vi "Periodic Message Generator.vi"(0 "J1939 Cluster":T4, 1 "Scale Ref":T2, 2 "Data Ref":T1, 5 "Output Array":T3[](array[typedef]) {"Identifier" format="%08x"}, 7 "Timeouts":T5[](array[typedef]) {"Arb ID" format="%.0x"}, 11 "error in":errorcluster) -> (4 "J1939 Cluster Out":T4, 6 "Output Array":T3[](array[typedef]) {"Identifier" format="%08x"}, 8 "Empty?":bool, 15 "error out":errorcluster)   [LabVIEW 2015, in "J1939 Addon Engine.lvlib"]
uses:
  J1939 Addon Engine.lvlib
  SubVIs/Periodic Message Generator Cluster.ctl
  Shared/J1939 Utilities/Types/CAN Outgoing Message Cluster.ctl
  Types/Setup Information Cluster.ctl
  <vilib>/xnet/xnet.llb/XNET Frame CAN.ctl
  <vilib>/xnet/xnet.llb/XNET Frame Type CAN.ctl
  Types/Conversion Lookup Table Reference.ctl
  Types/Data Lookup Table Reference.ctl
  Types/Datatable Lookup DVR.ctl
  Conversion Lookup Table Get Conversion Parameter.vi
  Data Lookup Table Get Signals (Range).vi
  <vilib>/xnet/xnet.llb/XNET Convert.vi
  <vilib>/xnet/xnet.llb/XNET Convert (Signal to Frame Raw).vi
  Data Lookup Table.vi
  Conversion Lookup Table.vi
  Shared/J1939 Utilities/J1939 Utilities.lvlib
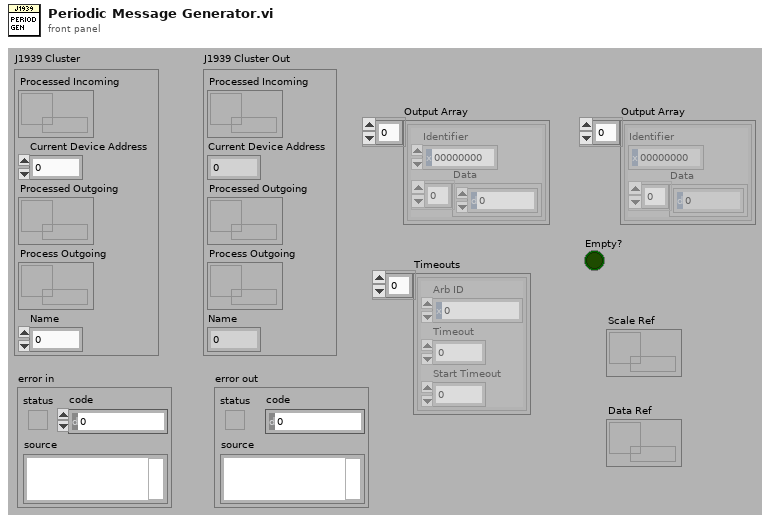
[diagram p1: front panel]
types:
  T1 = typedef "J1939 Addon Engine.lvlib/Data Lookup Table Reference.ctl" = refnum<data-value>
  T2 = typedef "J1939 Addon Engine.lvlib/Conversion Lookup Table Reference.ctl" = refnum<data-value>
  T3 = typedef "J1939 Addon Shared.lvlib/J1939 Utilities.lvlib/CAN Outgoing Message Cluster.ctl" = cluster{"Identifier":u32, "Data":u8[]}
  T4 = typedef "J1939 Addon Engine.lvlib/Setup Information Cluster.ctl" = cluster{"Processed Incoming":refnum<queue>, "Current Device Address":u8, "Processed Outgoing":refnum<queue>, "Process Outgoing":refnum<queue>, "Name":u64}
  T5 = typedef "J1939 Addon Engine.lvlib/Periodic Message Generator Cluster.ctl" = cluster{"Arb ID":u32, "Timeout":u32, "Start Timeout":u32}
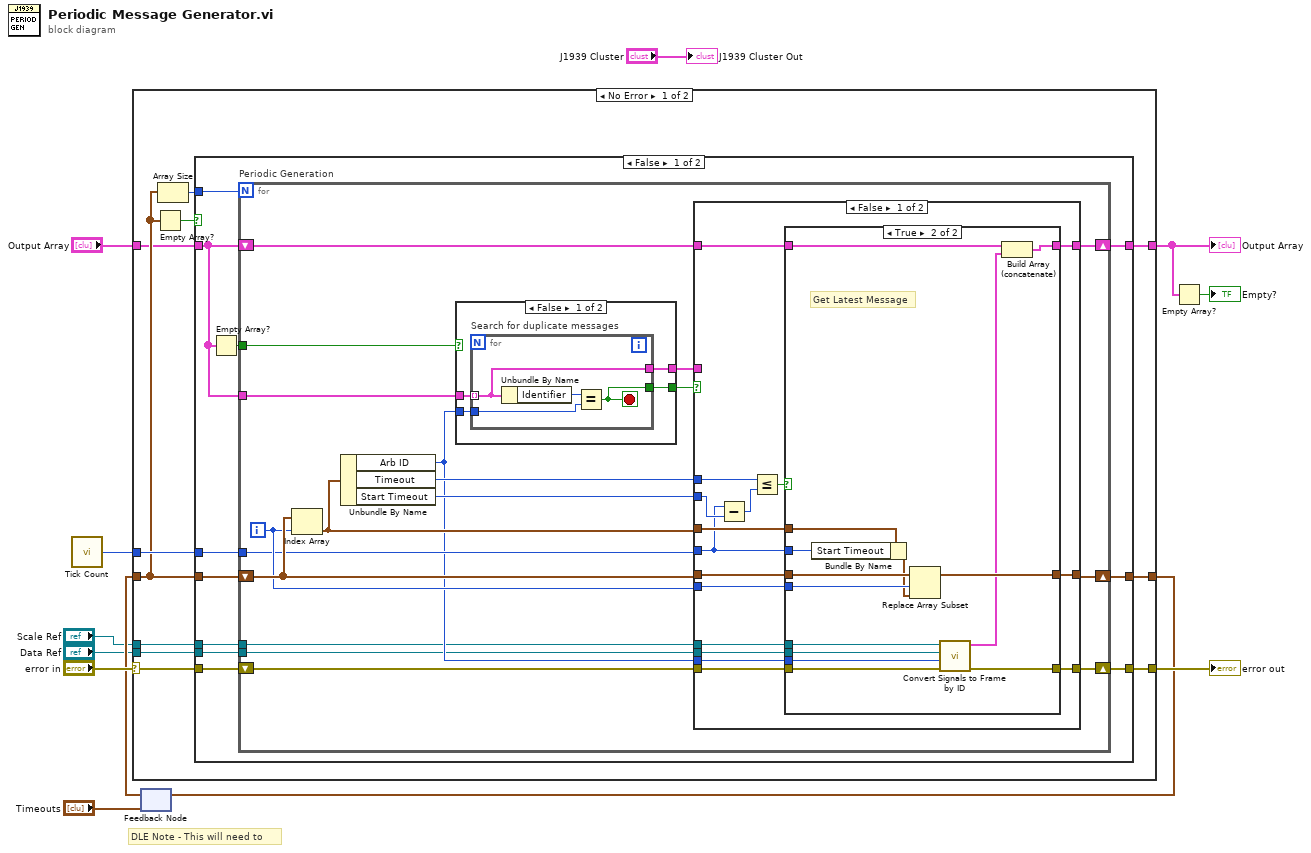
[diagram p0: block diagram]
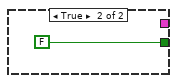
[diagram p2: hidden frame]
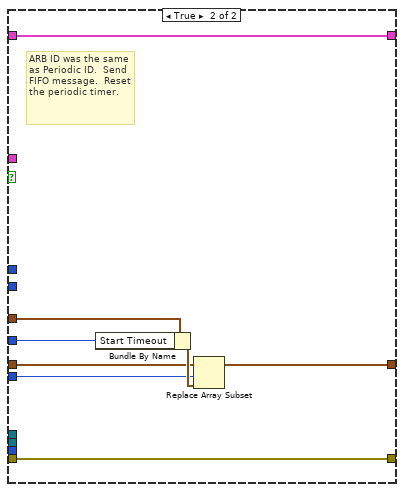
[diagram p4: hidden frame]
diagram:
  # "DLE Note - This will need to"
  n1 = call "Tick Count"() -> ("Tick Count(mSec)"=w10:u32)
  n2 = feedback #1("Timeouts") -> (w3:T5[])
  n3 = case shown="No Error" "error in" {
    selector: "error in" -> [w16 w108]
    tunnel: w3 -> [w20 w107]
    tunnel: [w22 w106] -> w6
    tunnel: [w15 w108] -> w11
    tunnel: w10 -> [w21 _]
    tunnel: [w18 w107] -> w9
    tunnel: "Output Array" -> [w17 w106]
    tunnel: "Scale Ref" -> [w14 _]
    tunnel: "Data Ref" -> [w13 _]
    frame No Error {
      n4 = Empty Array?(array=w20) -> (empty?=w19:bool)
      n5 = Array Size(array=w20) -> (size(s)=w23:i32)
      n6 = case shown="False" w19 {
        tunnel: w23 -> [w34 _]
        tunnel: [w30 w105] -> w22
        tunnel: w21 -> [w32 _]
        tunnel: w17 -> [w27 w105]
        tunnel: w20 -> [w33 w104]
        tunnel: [w31 w104] -> w18
        tunnel: w16 -> [w29 w103]
        tunnel: [w28 w103] -> w15
        tunnel: w14 -> [w25 _]
        tunnel: w13 -> [w24 _]
        frame False {
          n7 = Empty Array?(array=w27) -> (empty?=w26:bool)
          n8 = for "Periodic Generation" {
            N: w34 -> [_]
            tunnel: w32 -> [w44]
            shift-right: [w51] -> w30
            shift-left: w27 -> [w52]
            shift-right: [w48] -> w31
            shift-left: w33 -> [w49]
            tunnel: w27 -> [w45]
            shift-right: [w39] -> w28
            shift-left: w29 -> [w38]
            tunnel: w26 -> [w41]
            tunnel: w25 -> [w36]
            tunnel: w24 -> [w35]
            i -> [w47]
            n9 = Index Array(array=w49, index=w47) -> (element=w50:T5)
            n10 = Unbundle By Name(w50) -> ("Arb ID"=w37:u32, "Timeout"=w43:u32, "Start Timeout"=w42:u32)
            n11 = case shown="False" w41 {
              tunnel: [w56 FALSE] -> w46
              tunnel: w45 -> [w55 _]
              tunnel: w37 -> [w54 _]
              tunnel: [w53 _] -> w40
              frame False {
                n12 = for "Search for duplicate messages" {
                  tunnel: w55 -> [w57] mode=indexing
                  tunnel: w54 -> [w60]
                  tunnel: [w59] -> w56
                  tunnel: [w57] -> w53
                  stop <- w59 stop-if-true
                  n13 = Unbundle By Name(w57) -> ("Identifier"=w58:u32)
                  n14 = Equal?(x=w58, y=w60) -> (x = y?=w59:bool)
                }
              }
              frame True {
              }
            }
            n15 = case shown="False" w46 {
              tunnel: w52 -> [w77 w96]
              tunnel: [w76 w96] -> w51
              tunnel: w50 -> [w75 w100]
              tunnel: w44 -> [w69 w99]
              tunnel: w49 -> [w74 w101]
              tunnel: [w73 w97] -> w48
              tunnel: w47 -> [w72 w98]
              tunnel: w42 -> [w70 _]
              tunnel: w43 -> [w67 _]
              tunnel: w40 -> [_ _]
              tunnel: [w66 w95] -> w39
              tunnel: w38 -> [w65 w95]
              tunnel: w37 -> [w64 _]
              tunnel: w36 -> [w63 _]
              tunnel: w35 -> [w62 _]
              frame False {
                n16 = Subtract(x=w69, y=w70) -> (x-y=w71:u32)
                n17 = Less Or Equal?(x=w67, y=w71) -> (x <= y?=w68:bool)
                n18 = case shown="True" w68 {
                  tunnel: w77 -> [w80 w88]
                  tunnel: [w80 w87] -> w76
                  tunnel: w75 -> [_ w91]
                  tunnel: w69 -> [_ w89]
                  tunnel: w74 -> [w79 w94]
                  tunnel: [w79 w93] -> w73
                  tunnel: w72 -> [_ w92]
                  tunnel: [w78 w84] -> w66
                  tunnel: w65 -> [w78 w85]
                  tunnel: w64 -> [_ w83]
                  tunnel: w63 -> [_ w82]
                  tunnel: w62 -> [_ w81]
                  frame False {
                    # "Timeout has not expired"
                  }
                  frame True {
                    # "Get Latest Message"
                    n19 = Bundle By Name(cluster=w91, "Start Timeout"=w89) -> (w90:T5)
                    n20 = Replace Array Subset(array=w94, new element=w90, index=w92) -> (w93:T5[])
                    n21 = call "Convert Signals to Frame by ID.vi"("error in (no error)"=w85, "ID"=w83, "Data Ref"=w81, "Scale Ref"=w82) -> ("error out"=w84:errorcluster, "Frame"=w86:T3)  [unwired: 5 in, 1 out]
                    n22 = Build Array (concatenate)(w88, w86) -> (w87:T3[])
                  }
                }
              }
              frame True {
                # "ARB ID was the same as Periodic ID.  Send FIFO message.  Reset the periodic timer."
                n23 = Bundle By Name(cluster=w100, "Start Timeout"=w99) -> (w102:T5)
                n24 = Replace Array Subset(array=w101, new element=w102, index=w98) -> (w97:T5[])
              }
            }
          }
        }
        frame True {
          # "No periodic messages."
        }
      }
    }
    frame Error {
    }
  }
  "error out" <- w11
  "Output Array" <- w6
  n25 = feedback-in #1(w9) -> ()
  n26 = Empty Array?(array=w6) -> (empty?=→"Empty?":bool)
  "J1939 Cluster Out" <- "J1939 Cluster"
